vi "LaserLineDetection_Intensity_ExtendedSearch.vi"(0 "Image In":T1, 1 "Image Center (Horizontal)":i32, 2 "Search Distance":i32, 5 "slope In":dbl, 7 "intercept In":dbl, 9 "INTENSITYarray":u8[](array[numeric]), 11 "error in (no error)":errorcluster, 12 "Camera Parameters":T2) -> (4 "Image Out":T1, 6 "slope ES":dbl, 8 "intercept ES":dbl, 10 "appended array":cluster{u8[], i32[]}[][](array[cluster]), 14 "Extended Search Accepted":bool, 15 "error out":errorcluster)   [LabVIEW 2013]
uses:
  <vilib>/vision/Image Controls.llb/IMAQ Image.ctl
  Point Information.ctl
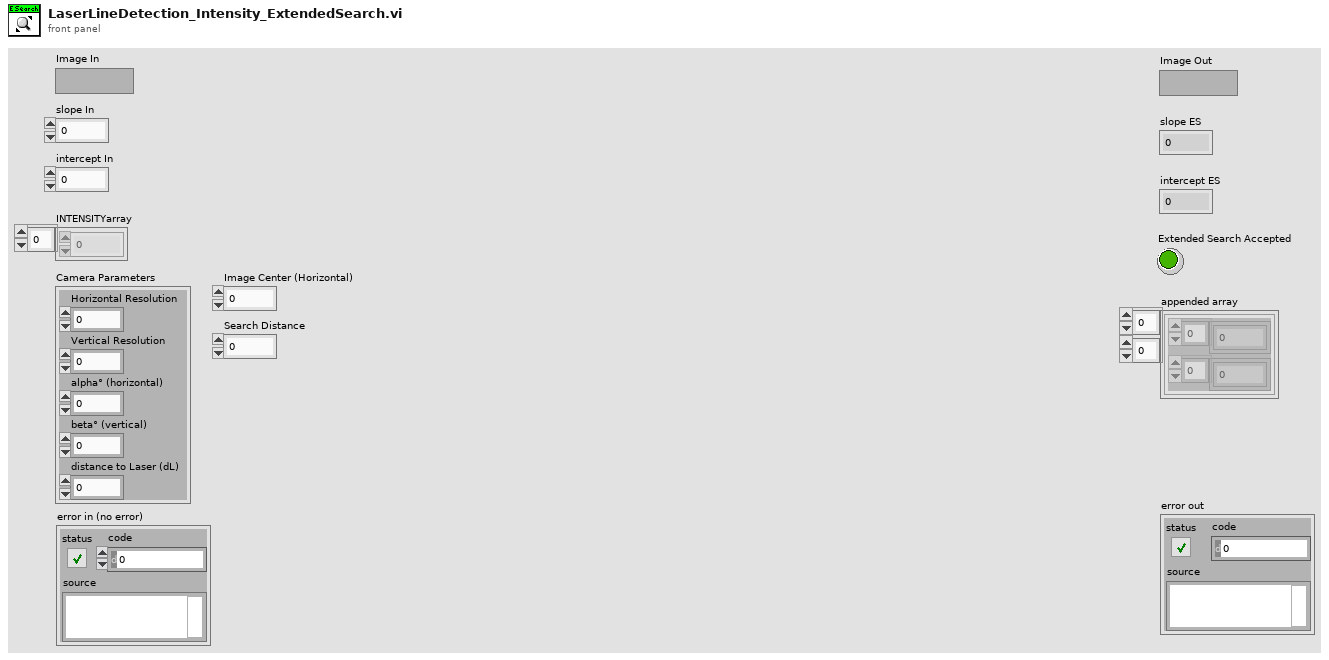
[diagram p1: front panel]
types:
  T1 = typedef "IMAQ Image.ctl" = refnum<image>
  T2 = cluster{"Horizontal Resolution":dbl, "Vertical Resolution":dbl, "alpha° (horizontal)":dbl, "beta° (vertical)":dbl, "distance to Laser (dL)":dbl}
  T3 = typedef "Point Information.ctl" = cluster{"X":i32, "Y":i32, "Intensity":u8}
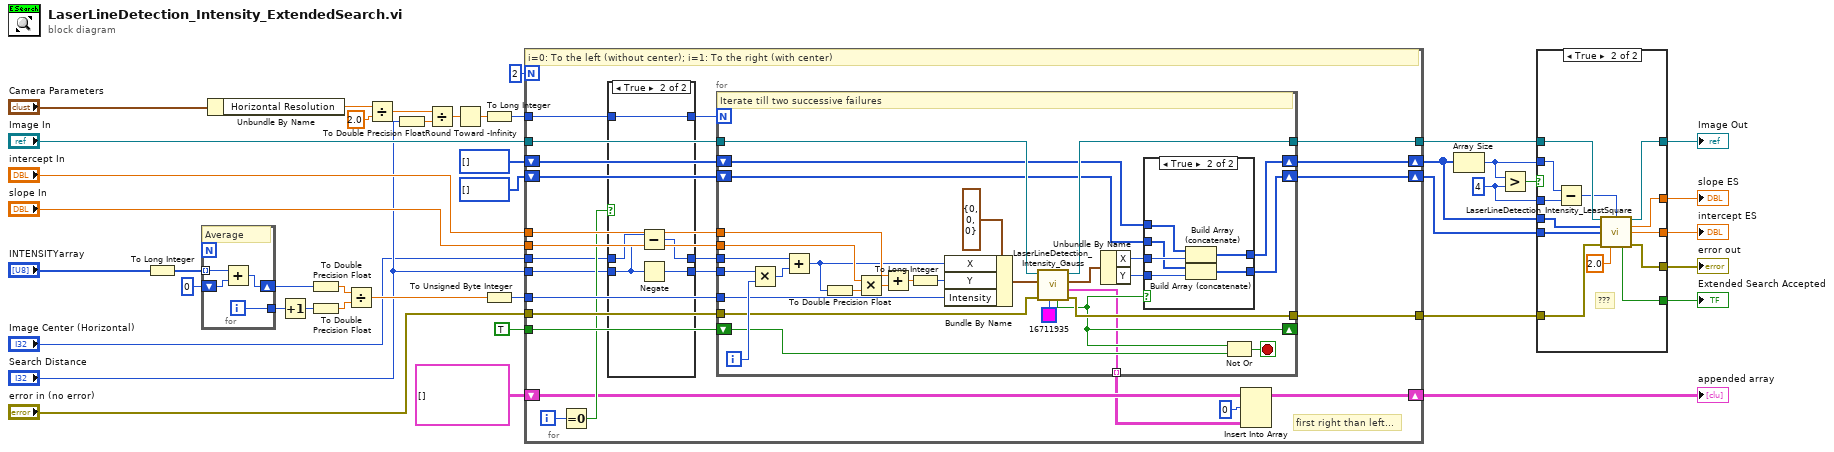
[diagram p0: block diagram]
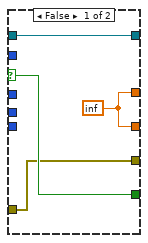
[diagram p2: hidden frame]
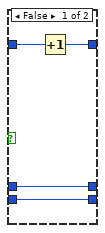
[diagram p3: hidden frame]
diagram:
  w3 = 4 ("y")
  n1 = To Long Integer(number="INTENSITYarray") -> (32bit integer=w28:i32[])
  n2 = for {
    tunnel: w28 -> [w46] mode=indexing
    shift-right: [w44] -> w30
    shift-left: 0 ("y") -> [w45]
    tunnel: [w43] -> w34
    i -> [w43]
    # "Average"
    n3 = Add(x=w46, y=w45) -> (x+y=w44:i32)
  }
  n4 = Unbundle By Name("Camera Parameters") -> ("Horizontal Resolution"=w37:dbl)
  n5 = Increment(x=w34) -> (x+1=w33:i32)
  n6 = To Double Precision Float(number=w30) -> (double precision float=w31:dbl)
  n7 = To Double Precision Float(number=w33) -> (double precision float=w32:dbl)
  n8 = Divide(x=w31, y=w32) -> (x/y=w35:dbl)
  n9 = Divide(x=w37, y=2.0) -> (x/y=w39:dbl)
  n10 = To Double Precision Float(number="Search Distance") -> (double precision float=w40:dbl)
  n11 = Divide(x=w39, y=w40) -> (x/y=w41:dbl)
  n12 = Round Toward -Infinity(1:w41) -> (0:w42:dbl)
  n13 = To Long Integer(number=w42) -> (32bit integer=w24:i32)
  n14 = To Unsigned Byte Integer(number=w35) -> (unsigned 8bit integer=w21:u8)
  n15 = for {
    N: 2 -> [_]
    tunnel: "error in (no error)" -> [w70]
    tunnel: "Image In" -> [w69]
    tunnel: w24 -> [w60]
    tunnel: [w68] -> w10
    tunnel: [w67] -> w11
    tunnel: "intercept In" -> [w66]
    tunnel: "slope In" -> [w65]
    tunnel: w21 -> [w64]
    tunnel: TRUE ("Gauss Fit Accepted") -> [w63]
    tunnel: "Search Distance" -> [w57]
    tunnel: "Image Center (Horizontal)" -> [w58]
    shift-right: [w54] -> w9
    shift-left: i32[] [] -> [w52]
    shift-right: [w53] -> w14
    shift-left: i32[] [] ("appended array") -> [w51]
    shift-right: [w49] -> w1
    shift-left: cluster{u8[], i32[]}[][] [] ("appended array") -> [w50]
    i -> [w62]
    # "first right than left..."
    # "i=0: To the left (without center); i=1: To the right (with center)"
    n16 = Equal To 0?(x=w62) -> (x = 0?=w61:bool)
    n17 = case shown="True" w61 {
      tunnel: w60 -> [w74 w79]
      tunnel: [w73 w79] -> w59
      tunnel: w58 -> [w72 w78]
      tunnel: w57 -> [w71 w76]
      tunnel: [w72 w77] -> w56
      tunnel: [w71 w75] -> w55
      frame False {
        n18 = Increment(x=w74) -> (x+1=w73:i32)
      }
      frame True {
        n19 = Subtract(x=w78, y=w76) -> (x-y=w77:i32)
        n20 = Negate(x=w76) -> (-x=w75:i32)
      }
    }
    n21 = for {
      N: w59 -> [_]
      tunnel: w55 -> [w107]
      tunnel: w56 -> [w106]
      tunnel: w69 -> [w104]
      tunnel: [w103] -> w67
      tunnel: w70 -> [w102]
      tunnel: [w101] -> w68
      tunnel: w65 -> [w97]
      tunnel: w66 -> [w96]
      shift-right: [w88] -> _
      shift-left: w63 -> [w90]
      tunnel: w64 -> [w89]
      shift-right: [w84] -> w54
      shift-left: w52 -> [w82]
      shift-right: [w83] -> w53
      shift-left: w51 -> [w81]
      tunnel: [w80] -> w48 mode=indexing
      i -> [w108]
      stop <- w91 stop-if-true
      # "Iterate till two successive failures"
      n22 = Multiply(x=w107, y=w108) -> (x*y=w109:i32)
      n23 = Add(x=w106, y=w109) -> (x+y=w93:i32)
      n24 = To Double Precision Float(number=w93) -> (double precision float=w92:dbl)
      n25 = Multiply(x=w97, y=w92) -> (x*y=w98:dbl)
      n26 = Add(x=w96, y=w98) -> (x+y=w95:dbl)
      n27 = To Long Integer(number=w95) -> (32bit integer=w94:i32)
      n28 = Bundle By Name(cluster=T3 {"X"=0, "Y"=0, "Intensity"=0} ("Point Information In"), "X"=w93, "Y"=w94, "Intensity"=w89) -> (w99:T3)
      n29 = call "LaserLineDetection_Intensity_Gauss.vi"("Color"=u32 16711935, "Error In"=w102, "Point Information In"=w99, "Source In"=w104) -> ("Error Out"=w101:errorcluster, "appended array"=w80:cluster{u8[], i32[]}[], "Point Information Out"=w87:T3, "Source Out"=w103:T1, "Gauss Fit Accepted"=w88:bool)  [unwired: 2 in, 1 out]
      n30 = Unbundle By Name(w87) -> ("X"=w86:i32, "Y"=w85:i32)
      n31 = case shown="True" w88 {
        tunnel: w86 -> [_ w117]
        tunnel: w85 -> [_ w116]
        tunnel: [w111 w115] -> w84
        tunnel: [w110 w114] -> w83
        tunnel: w82 -> [w111 w113]
        tunnel: w81 -> [w110 w112]
        frame False {
        }
        frame True {
          n32 = Build Array (concatenate)(w113, w117) -> (w115:i32[])
          n33 = Build Array (concatenate)(w112, w116) -> (w114:i32[])
        }
      }
      n34 = Not Or(1:w90, 2:w88) -> (0:w91:bool)
    }
    n35 = Insert Into Array(array=w50, index (row)=0, new element=w48) -> (w49:cluster{u8[], i32[]}[][])  [unwired: 1 in]
  }
  "appended array" <- w1
  n36 = Array Size(array=w9) -> (size(s)=w8:i32)
  n37 = Greater?(x=w8, y=w3) -> (0:w7:bool)
  n38 = case shown="True" w7 {
    selector: w7 -> [w121 _]
    tunnel: [w119 w134] -> w16
    tunnel: [w120 w133] -> w15
    tunnel: w14 -> [_ w132]
    tunnel: w11 -> [w120 w131]
    tunnel: w10 -> [w119 w130]
    tunnel: w9 -> [_ w129]
    tunnel: w8 -> [_ w127]
    tunnel: [w121 w126] -> w6
    tunnel: [w118 w125] -> w5
    tunnel: [w118 w124] -> w4
    tunnel: w3 -> [_ w123]
    frame False {
      w118 = inf
    }
    frame True {
      # "???"
      n39 = Subtract(x=w127, y=w123) -> (x-y=w122:i32)
      n40 = call "LaserLineDetection_Intensity_LeastSquare.vi"("Image In"=w131, "Loop Count"=w122, "Xarray In"=w129, "Yarray In"=w132, "error in (no error)"=w130, "tolerance (residue)"=2.0) -> ("Image Out"=w133:T1, "slope"=w125:dbl, "intercept"=w124:dbl, "Least Square Accepted"=w126:bool, "error out"=w134:errorcluster)  [unwired: 2 in, 3 out]
    }
  }
  "Image Out" <- w15
  "error out" <- w16
  "Extended Search Accepted" <- w6
  "slope ES" <- w5
  "intercept ES" <- w4
